vi "dll.midi_file_open.vi"(8 "error in (no error)":errorcluster, 10 "MIDI File":path, 11 "midi file in":refnum<class "midi file.lvclass">) -> (0 "error out":errorcluster, 3 "midi file out":refnum<class "midi file.lvclass">)   [LabVIEW 2020, in "MIDIllan.lvlib" / "midi file.lvclass"]
uses:
  midi file.lvclass
  midi file.lvclass/midi file.ctl
  MIDIllan/MIDIllan.lvlib
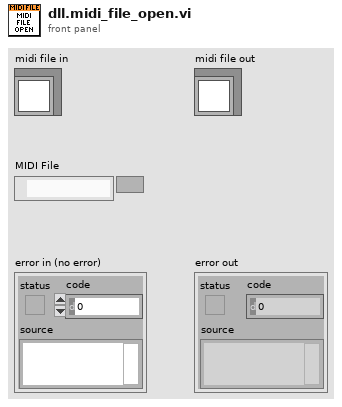
[diagram p1: front panel]
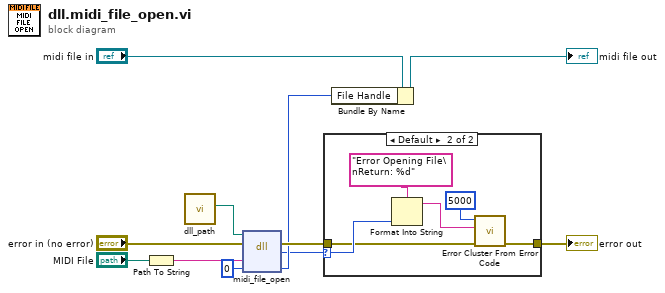
[diagram p0: block diagram]
diagram:
  n1 = Path To String(path="MIDI File") -> (string=w9:string)
  n2 = call "dll_path.vi"() -> ("dll"=w11:path)  [unwired: 11 in]
  n3 = dll-call lib="C:/code/LabVIEW-MIDI-XPLAT/dist/TomMIDIllan_*.*" fn="midi_file_open"(path in=w11, error in="error in (no error)", "File Path"=w9, "File Handle"=0) -> (error out=w5:errorcluster, "Error code"=w2:i32, "File Handle"=w3:i32)  [unwired: 2 in, 1 out]
  n4 = case shown="Default" w2 {
    selector: w2 -> [_ w15]
    tunnel: w5 -> [w12 w14]
    tunnel: [w12 w13] -> w4
    frame 0.. {
    }
    frame Default {
      n5 = Format Into String(format string="Error Opening File\nReturn: %d", w15) -> (resulting string=w16:string)  [unwired: 2 in, 1 out]
      n6 = call <vilib>:"Error Cluster From Error Code.vi"("error in (no error)"=w14, "error message (\"\")"=w16, "error code (0)"=5000) -> ("error out"=w13:errorcluster)  [unwired: 6 in]
    }
  }
  "error out" <- w4
  n7 = Bundle By Name(cluster="midi file in", "File Handle"=w3) -> (→"midi file out":refnum<class "midi file.lvclass">)
